vi "exercise 5-3.vi"() -> ()   [LabVIEW 2014]
uses:
  type def numeric.ctl
  def numeric.ctl
panel:
  in  "Strict Type Def Numeric 2":dbl
  in  "Type Def Numeric":T1
  in  "Strict Type Def Numeric":T2
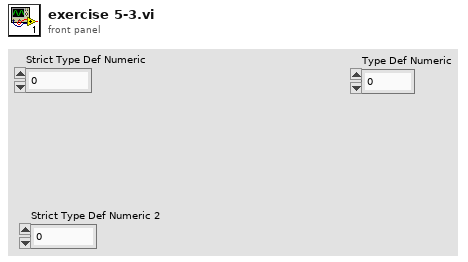
[diagram p1: front panel]
types:
  T1 = typedef "def numeric.ctl" = dbl
  T2 = typedef "type def numeric.ctl" = dbl
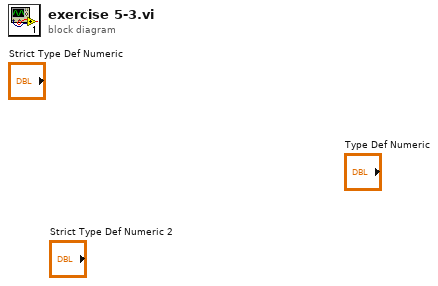
[diagram p0: block diagram]
diagram:
